vi "Get Sender.vi"(11 "No Op Msg in":refnum<class "No Op Msg.lvclass">) -> (2 "Sender":refnum<class "Sender.lvclass">)   [LabVIEW 2020, in "jettl.lvlib" / "No Op Msg.lvlib" / "No Op Msg.lvclass"]
uses:
  No Op Msg.lvclass
  Sender/Sender/Sender.lvclass
  No Op Msg.lvclass/No Op Msg.ctl
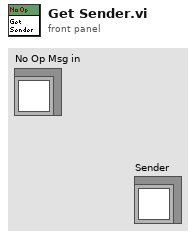
[diagram p1: front panel]
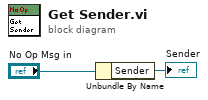
[diagram p0: block diagram]
diagram:
  n1 = Unbundle By Name("No Op Msg in") -> ("Sender"=→"Sender":refnum<class "Sender.lvclass">)
